vi "Write String Direct.vi"(8 "error in (no error)":errorcluster, 9 "Timeout (ms)":i32, 10 "Data":string, 11 "CIFTag in":refnum<class "CIF_CIPC_Chn_String.lvclass">) -> (0 "error out":errorcluster, 1 "timed out?":bool, 3 "CIFTag out":refnum<class "CIF_CIPC_Chn_String.lvclass">)   [LabVIEW 2021, in "CIF_CIPC_Chn_String.lvclass"]
uses:
  CIF_CIPC_Chn_String.lvclass
  D:/dev/Packages/CIF_Channels_Core/src/CIFChannels/CIFChannels.lvclass
  D:/dev/Packages/CIF_Channels_Core/src/CIPC_Channels/CIF_CIPC_Chan/CIF_CIPC_Chn.lvclass
  CIFChannels/CIFChannels.lvclass/CIFChannels.ctl
  CIF_CIPC_Chan/CIF_CIPC_Chn.lvclass/CIF_CIPC_Chn.ctl
  CIF_CIPC_Chn_String.lvclass/CIF_CIPC_Chn_String.ctl
  ChannelCommon/typedef/Errors.ctl
  4dec1408-e4ff-48ac-a735-b713bf84484a.vi
  CIFChannels/Accessors/Read Tag Forced.vi
  <vilib>/CIF Foundation/CIF CIPC/SubVIs/Check Error.vi
  <vilib>/CIF Foundation/CIF CIPC/SubVIs/Get dll Path.vi
  <vilib>/CIF Foundation/CIF CIPC/SubVIs/Notify Of New Write.vi
  <vilib>/CIF Foundation/CIF CIPC/SubVIs/Get Element Write Position.vi
  <vilib>/CIF Foundation/CIF Utilities/Errors/Append Error Location.vi
  <vilib>/CIF Foundation/CIF CIPC/SubVIs/Get Element Info Variant.vi
  <vilib>/Utility/error.llb/Trim Whitespace.vi
  <vilib>/Utility/error.llb/Error Cluster From Error Code.vi
  CIF_CIPC_Chan/CIF_CIPC_Chn.lvclass
  ChannelCommon/ChannelCommon.lvlib
  D:/dev/Packages/CIF_Channels_Core/src/CIPC_Channels/String/CIF_CIPC_Chn_String.lvclass
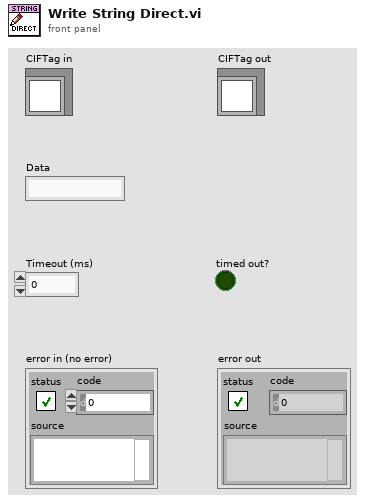
[diagram p1: front panel]
types:
  T1 = typedef "ChannelCommon.lvlib/Errors.ctl" = enum16{"gRPC Server Not Found", "Duplicate Channel", "Missing Channel", "Incorrect Type", "Flatten Error", "Unflatten Data", "Channel Length", "Plugin Connection", "gRPC Server Connection", "FIFO Unflatten", "Required Override", "Remove Not Found", "Multi Sub Not Supported", "Primary Already Connected", "Backpressure Not Supported", "Unable to Increase Buffer", "Data too Large"}
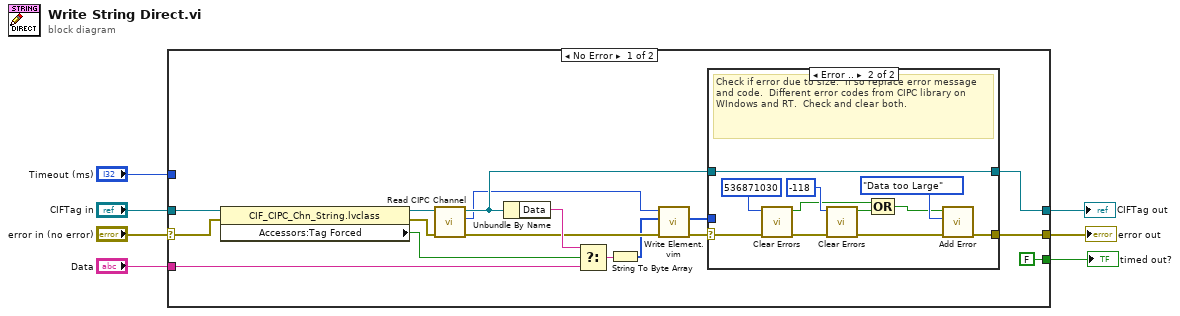
[diagram p0: block diagram]
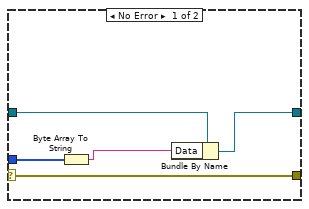
[diagram p2: hidden frame]
diagram:
  n1 = case shown="No Error" "error in (no error)" {
    selector: "error in (no error)" -> [w23 w42]
    tunnel: [w8 w42] -> w2
    tunnel: [w13 w41] -> w3
    tunnel: "CIFTag in" -> [w24 w41]
    tunnel: "Data" -> [w21 _]
    tunnel: [FALSE ("Timed out?") _] -> w1
    tunnel: "Timeout (ms)" -> [_ _]
    frame No Error {
      n2 = property class="CIF_CIPC_Chn_String.lvclass"(reference=w24, error in=w23) -> (reference out=w19:refnum<class "CIF_CIPC_Chn_String.lvclass">, error out=w18:errorcluster, "Accessors:Tag Forced"=w22:bool)
      n3 = call "Read CIPC Channel.vi"("error in (no error)"=w18, "CIFTag in"=w19) -> ("error out"=w16:errorcluster, "CIPC Channel"=w15:u64, "CIFTag out"=w17:refnum<class "CIF_CIPC_Chn_String.lvclass">)  [unwired: 7 in]
      n4 = Unbundle By Name(w17) -> ("Data"=w20:string)
      n5 = Select(t=w20, s=w22, f=w21) -> (s? t:f=w14:string)
      n6 = String To Byte Array(string=w14) -> (unsigned byte array=w10:u8[])
      n7 = call "Write Element.vim"("error in (no error)"=w16, "Data in"=w10, "CIPC Reference in"=w15) -> ("error out"=w9:errorcluster, "Data out"=w12:u8[])  [unwired: 5 in, 2 out]
      n8 = case shown="Error .." w9 {
        selector: w9 -> [w25 w36]
        tunnel: w17 -> [w29 w40]
        tunnel: [w28 w40] -> w13
        tunnel: w12 -> [w27 _]
        tunnel: [w25 w38] -> w8
        frame No Error {
          n9 = Byte Array To String(unsigned byte array=w27) -> (string=w26:string)
          n10 = Bundle By Name(cluster=w29, "Data"=w26) -> (w28:refnum<class "CIF_CIPC_Chn_String.lvclass">)
        }
        frame Error {
          # "Check if error due to size.  If so replace error message and code.  Different error codes from CIPC library on WIndows and RT.  Check and clear both."
          n11 = call <vilib>:"Clear Errors.vi"("error in (no error)"=w36, "specific error code to clear (0: all)"=536871030) -> ("error out"=w35:errorcluster, "specific error cleared?"=w32:bool)  [unwired: 4 in]
          n12 = call <vilib>:"Clear Errors.vi"("error in (no error)"=w35, "specific error code to clear (0: all)"=-118) -> ("error out"=w30:errorcluster, "specific error cleared?"=w33:bool)  [unwired: 4 in]
          n13 = Compound Arithmetic op=OR(w32, w33) -> (w31:bool)
          n14 = call "Add Error.vi"("error in (no error)"=w30, "Error"=Errors."Data too Large", "Insert Error"=w31) -> ("error out"=w38:errorcluster)  [unwired: 8 in]
        }
      }
    }
    frame Error {
    }
  }
  "error out" <- w2
  "CIFTag out" <- w3
  "timed out?" <- w1
